vi "Remove Helper Extension from Hierarchy.vi"(11 "Hierarchy":string[](array[string])) -> (3 "Hierarchy without Helper Extensions":string[](array[string]))   [LabVIEW 2020, in "VI Properties Editor.lvlib" / "Project Tree Map.lvclass"]
uses:
  Project Tree Map.lvclass
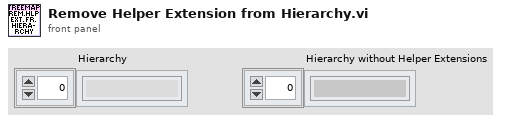
[diagram p1: front panel]
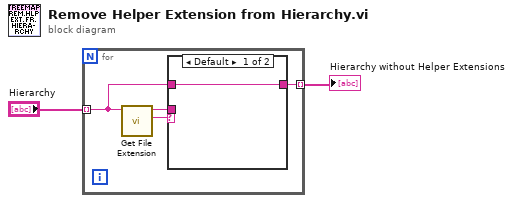
[diagram p0: block diagram]
diagram:
  n1 = for {
    tunnel: [w4] -> w1 mode=indexing
    tunnel: "Hierarchy" -> [w3] mode=indexing
    n2 = call "Get File Extension.vi"("Filename"=w3) -> ("Lowercase Extension"=w6:string, "Filename without Extension"=w5:string)  [unwired: 9 in]
    n3 = case shown="Default" w6 {
      tunnel: w5 -> [_ w8]
      tunnel: w3 -> [w7 _]
      tunnel: [w7 w8] -> w4
      frame Default {
      }
      frame "target", "virtual" {
      }
    }
  }
  "Hierarchy without Helper Extensions" <- w1
